vi "All Data for Triggers.vi"(6 "input valid":bool, 9 "channel index":u8, 10 "data in":T1, 11 "reset":bool) -> (2 "output valid":bool, 3 "channel out":fxp<+/-,18,1>[](array[numeric]))   [LabVIEW 2021]
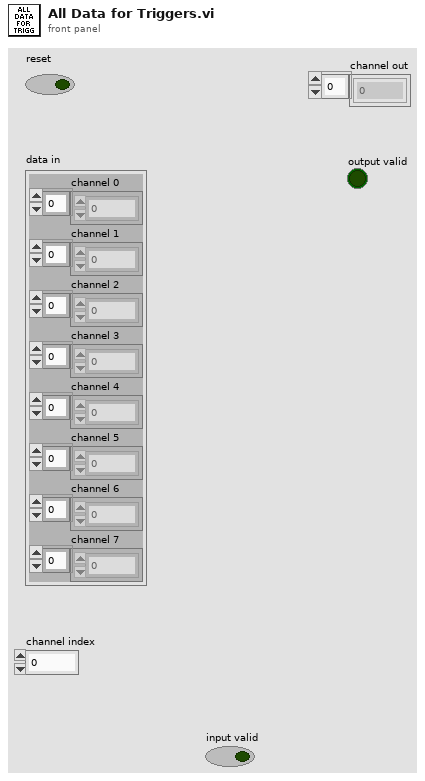
[diagram p1: front panel]
types:
  T1 = cluster{"channel 0":fxp<+/-,18,1>[], "channel 1":fxp<+/-,18,1>[], "channel 2":fxp<+/-,18,1>[], "channel 3":fxp<+/-,18,1>[], "channel 4":fxp<+/-,18,1>[], "channel 5":fxp<+/-,18,1>[], "channel 6":fxp<+/-,18,1>[], "channel 7":fxp<+/-,18,1>[]}
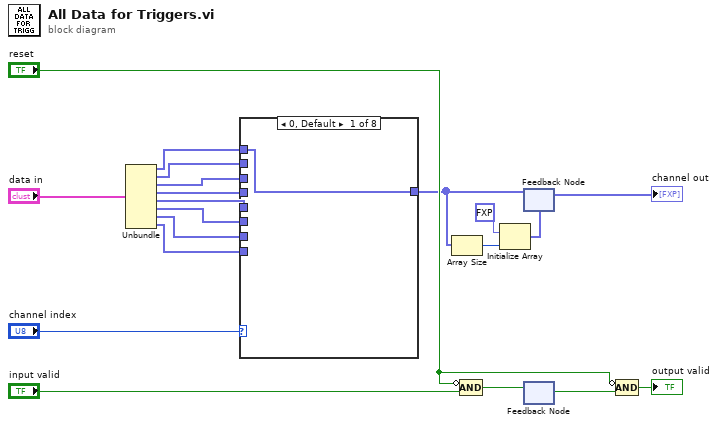
[diagram p0: block diagram]
diagram:
  n1 = Unbundle("data in") -> ("channel 0"=w2:fxp<+/-,18,1>[], "channel 1"=w3:fxp<+/-,18,1>[], "channel 2"=w4:fxp<+/-,18,1>[], "channel 3"=w5:fxp<+/-,18,1>[], "channel 4"=w6:fxp<+/-,18,1>[], "channel 5"=w7:fxp<+/-,18,1>[], "channel 6"=w8:fxp<+/-,18,1>[], "channel 7"=w9:fxp<+/-,18,1>[])
  n2 = case shown="0, Default" "channel index" {
    tunnel: w2 -> [w21 _ _ _ _ _ _ _]
    tunnel: w3 -> [_ w22 _ _ _ _ _ _]
    tunnel: [w21 w22 w23 w24 w25 w26 w27 w28] -> w13
    tunnel: w4 -> [_ _ w23 _ _ _ _ _]
    tunnel: w5 -> [_ _ _ w24 _ _ _ _]
    tunnel: w6 -> [_ _ _ _ w25 _ _ _]
    tunnel: w7 -> [_ _ _ _ _ w26 _ _]
    tunnel: w8 -> [_ _ _ _ _ _ w27 _]
    tunnel: w9 -> [_ _ _ _ _ _ _ w28]
    frame 0, Default {
    }
    frame 1 {
    }
    frame 2 {
    }
    frame 3 {
    }
    frame 4 {
    }
    frame 5 {
    }
    frame 6 {
    }
    frame 7 {
    }
  }
  n3 = Array Size(array=w13) -> (size(s)=w12:i32)
  n4 = Compound Arithmetic op=AND(invert "reset", "input valid") -> (w14:bool)
  n5 = Initialize Array(fxp<+/-,18,1> 0.0 ("Numeric"), w12) -> (w10:fxp<+/-,18,1>[])
  n6 = feedback #1(w10) -> (→"channel out":fxp<+/-,18,1>[])
  n7 = feedback-in #1(w13) -> ()
  n8 = feedback #2() -> (w16:bool)  [unwired: 1 in]
  n9 = feedback-in #2(w14) -> ()
  n10 = Compound Arithmetic op=AND(invert "reset", w16) -> (→"output valid":bool)
